vi "Graphics-Sort XY Graph (polymorphic).vi"   [LabVIEW 2020]
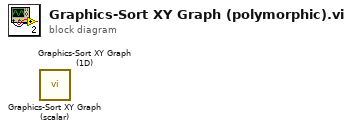
[diagram p0: block diagram]
diagram:
  n1 = call "Graphics-Sort XY Graph (scalar).vi"() -> ()  [unwired: 15 in, 1 out]
  n2 = call "Graphics-Sort XY Graph (1D).vi"() -> ()  [unwired: 15 in, 1 out]
